vi "Test_connect_and_ID.vi"() -> ()   [LabVIEW 2024]
uses:
  D:/A.C.M/Example CSharp_64/bin/Debug/Interop.DX10SDKADAPTORLib.dll
  Example CSharp_64/bin/Debug/Interop.DX10SDKADAPTORLib.dll
panel:
  out "ToString":string
  out "pbstrSerNum":string
  out "Connect":bool
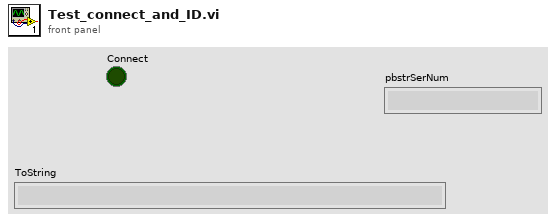
[diagram p1: front panel]
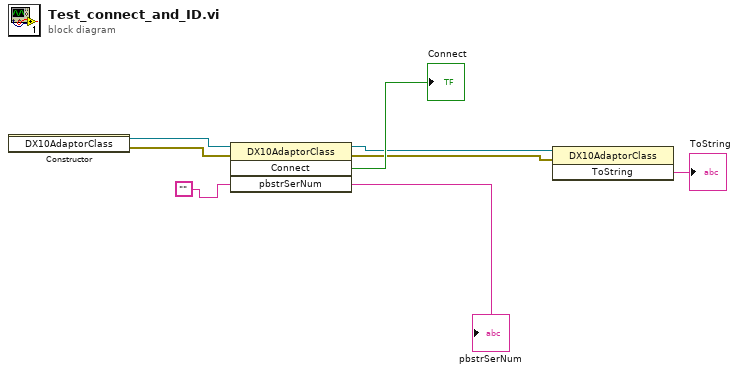
[diagram p0: block diagram]
diagram:
  n1 = constructor class="DX10AdaptorClass"() -> (reference out=w8:refnum<k24>, error out=w7:errorcluster)  [unwired: 3 in, 1 out]
  n2 = invoke class="DX10AdaptorClass" method="Connect"(reference=w8, error in=w7, "pbstrSerNum"="") -> (reference out=w3:refnum<k24>, error out=w2:errorcluster, "Connect"=→"Connect":bool, "pbstrSerNum"=→"pbstrSerNum":string)  [unwired: 1 in]
  n3 = invoke class="DX10AdaptorClass" method="ToString"(reference=w3, error in=w2) -> ("ToString"=→"ToString":string)  [unwired: 1 in, 2 out]
